vi "Add Attribute - 1D Array DBL.vi"(8 "error in (no error)":errorcluster, 9 "Value":dbl[](array[numeric]) caption="Value (empty)", 10 "Attribute":string, 11 "YAML Parser in":refnum<class "YAML Parser.lvclass">) -> (0 "error out":errorcluster, 3 "YAML Parser out":refnum<class "YAML Parser.lvclass">)   [LabVIEW 2015, in "YAML Parser.lvclass"]
uses:
  YAML Parser.lvclass
  YAML Parser.lvclass/YAML Parser.ctl
panel:
  out "replaced":bool
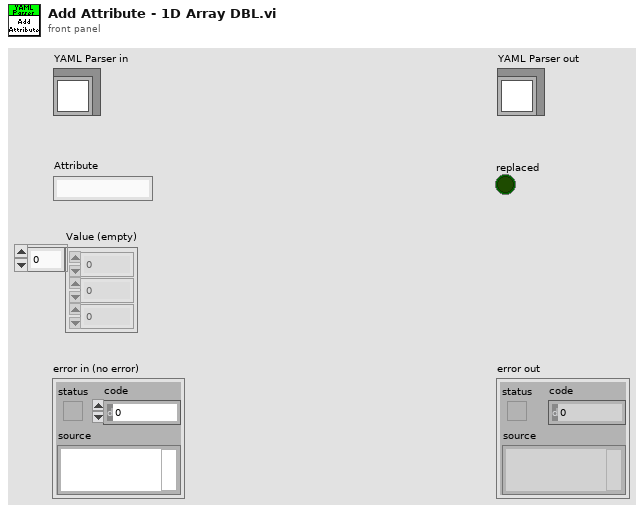
[diagram p1: front panel]
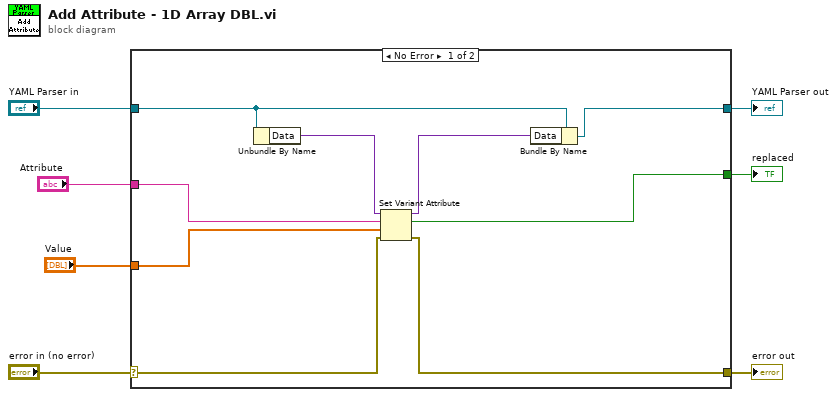
[diagram p0: block diagram]
diagram:
  n1 = case shown="No Error" "error in (no error)" {
    selector: "error in (no error)" -> [w14 w18]
    tunnel: [w13 w18] -> w6
    tunnel: [w16 w17] -> w4
    tunnel: "YAML Parser in" -> [w15 w17]
    tunnel: "Attribute" -> [w10 _]
    tunnel: "Value" -> [w9 _]
    tunnel: [w8 _] -> w1
    frame No Error {
      n2 = Unbundle By Name(w15) -> ("Data"=w12:variant)
      n3 = Set Variant Attribute(Variant=w12, name=w10, value=w9, error in=w14) -> (Variant out=w11:variant, replaced=w8:bool, error out=w13:errorcluster)
      n4 = Bundle By Name(cluster=w15, "Data"=w11) -> (w16:refnum<class "YAML Parser.lvclass">)
    }
    frame Error {
    }
  }
  "error out" <- w6
  "YAML Parser out" <- w4
  "replaced" <- w1
